vi "GDC Befehl senden.vi"(8 "error in (no error)":errorcluster caption="Fehler (Eingang, kein Fehler)", 9 "Daten":string[](array[string]), 10 "Befehl":string, 11 "VISA-Ressourcenname":refnum<visa-resource-name>) -> (0 "error out":errorcluster caption="Fehler (Ausgang)", 3 "VISA-Ressourcenname (Ausgang)":refnum<visa-resource-name>)   [LabVIEW 2020, in "Linearisierung v2.lvlib" / "Gasteiler.lvlib" / "Horiba GDC.lvlib"]
uses:
  Horiba GDC.lvlib
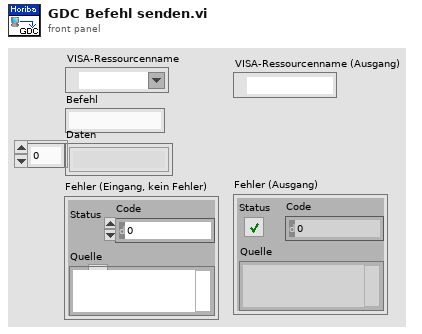
[diagram p1: front panel]
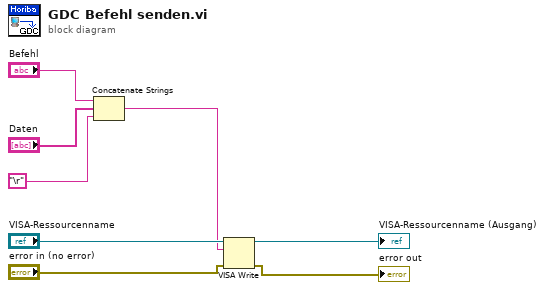
[diagram p0: block diagram]
diagram:
  n1 = Concatenate Strings("Befehl", "Daten", "\r") -> (w2:string)
  n2 = VISA Write(VISA resource name="VISA-Ressourcenname", write buffer=w2, error in (no error)="error in (no error)") -> (VISA resource name out=→"VISA-Ressourcenname (Ausgang)":refnum<visa-resource-name>, error out=→"error out":errorcluster)  [unwired: 1 out]
